vi "_get_fast_cmd_settings.vi"(7 "Settings in":string) -> (0 "*WAI":bool, 1 "OPC?":bool, 2 "ErrorCheckMode":i32, 3 "DataType":i32)   [LabVIEW 2020, in "Rohde&Schwarz RTx Oscilloscopes.lvlib" / "rsidr_core.lvlib"]
uses:
  rsidr_core.lvlib
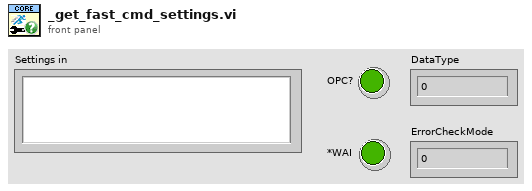
[diagram p1: front panel]
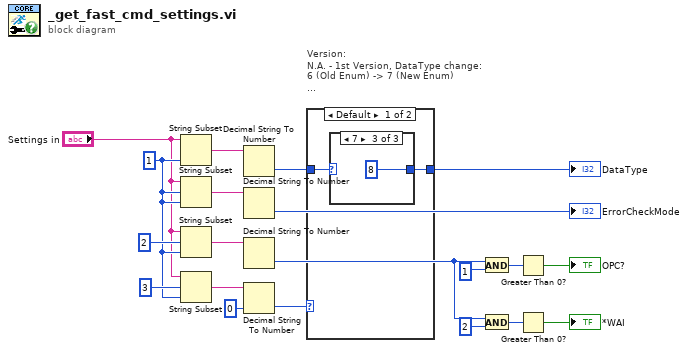
[diagram p0: block diagram]
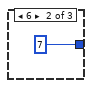
[diagram p3: hidden frame]
diagram:
  w7 = 1 ("length (rest)")
  n1 = String Subset(string="Settings in", length (rest)=w7) -> (substring=w20:string)  [unwired: 1 in]
  n2 = String Subset(string="Settings in", offset (0)=w7, length (rest)=w7) -> (substring=w19:string)
  n3 = String Subset(string="Settings in", offset (0)=2, length (rest)=w7) -> (substring=w17:string)
  n4 = String Subset(string="Settings in", offset (0)=3, length (rest)=w7) -> (substring=w5:string)
  n5 = Decimal String To Number(string=w20) -> (number=w2:i32)  [unwired: 2 in, 1 out]
  n6 = Decimal String To Number(string=w19) -> (number=→"ErrorCheckMode":i32)  [unwired: 2 in, 1 out]
  n7 = Decimal String To Number(string=w17) -> (number=w9:i32)  [unwired: 2 in, 1 out]
  n8 = Decimal String To Number(string=w5, default (0L)=0 ("default (0 I32)")) -> (number=w4:i32)  [unwired: 1 in, 1 out]
  n9 = case "Version:\nN.A. - 1st Version, DataType change:\n6 (Old Enum) -> 7 (New Enum)\n\n2 - 2nd Version, DataType is OK" shown="Default" w4 {
    tunnel: w2 -> [w22 w26]
    tunnel: [w21 w26] -> w1
    frame Default {
      n10 = case shown="7" w22 {
        selector: w22 -> [w23 _ _]
        tunnel: [w23 7 8] -> w21
        frame Default {
        }
        frame 6 {
        }
        frame 7 {
        }
      }
    }
    frame 2 {
    }
  }
  "DataType" <- w1
  n11 = And(x=w9, y=1) -> (x .and. y?=w14:i32)
  n12 = And(x=w9, y=2) -> (x .and. y?=w12:i32)
  n13 = Greater Than 0?(x=w14) -> (x > 0?=→"OPC?":bool)
  n14 = Greater Than 0?(x=w12) -> (x > 0?=→"*WAI":bool)
